vi "ABB Test No Load.vi"() -> ()   [LabVIEW 2017]
uses:
  Temp error msg.ctl
  Video Display Buttons.ctl
  <vilib>/Analysis/baseanly.llb/Mean (DBL).vi
  ABB global.vi
  <vilib>/Analysis/NI_AALPro.lvlib
  <vilib>/Analysis/NI_AALBase.lvlib
panel:
  in  "Video Displays":T1
  in  "Temp error":T2="Error: Temperature measurement "
  in  "Case Constant\n(See Context Help)":i32
  in  "Additional Mech Loss (kW)":dbl
  in  "show fit":bool
  out "Additional Temperatures  (°C)":string[][](table)
  in  "Simulate volts":dbl(slide) max=1800.0
  out "Temperatures  (°C)":string[][](table)
  out "Losses (kW)":string[][](table)
  out "Auto Readings":cluster{"%":dbl[], "Recorded":bool[]}
  out "In Range?":bool[](array[boolean])
  out "saved Readings":dbl[][](array[numeric])
  out "% rated voltage":dbl format="%.1f"
  out "Rated Volts":dbl
  out "Serial number":string
  out "W.O number":string
  out "Power":string[][](table)
  out "Voltage":string[][](table)
  out "Current":string[][](table)
  out "Norma 5000 Error":string
  in  "Record":bool
  out "Readings":string[][](table)
  in  "View":enum16{"Graph", "Readings"}(ring)
  out "Number readings":i32
  out "Status":enum16{"Stopped", "Running"}(ring)
  out "Timedate":string
  in  "End test":bool
  in  "Start":bool
  in  "Read Mode":enum16{"Auto", "Manual"}(ring)
  in  "Exit":bool
  out "Separation of losses":cluster{dbl[], "Best Linear Fit":dbl[]}[](graph)
  # "No Load Test"
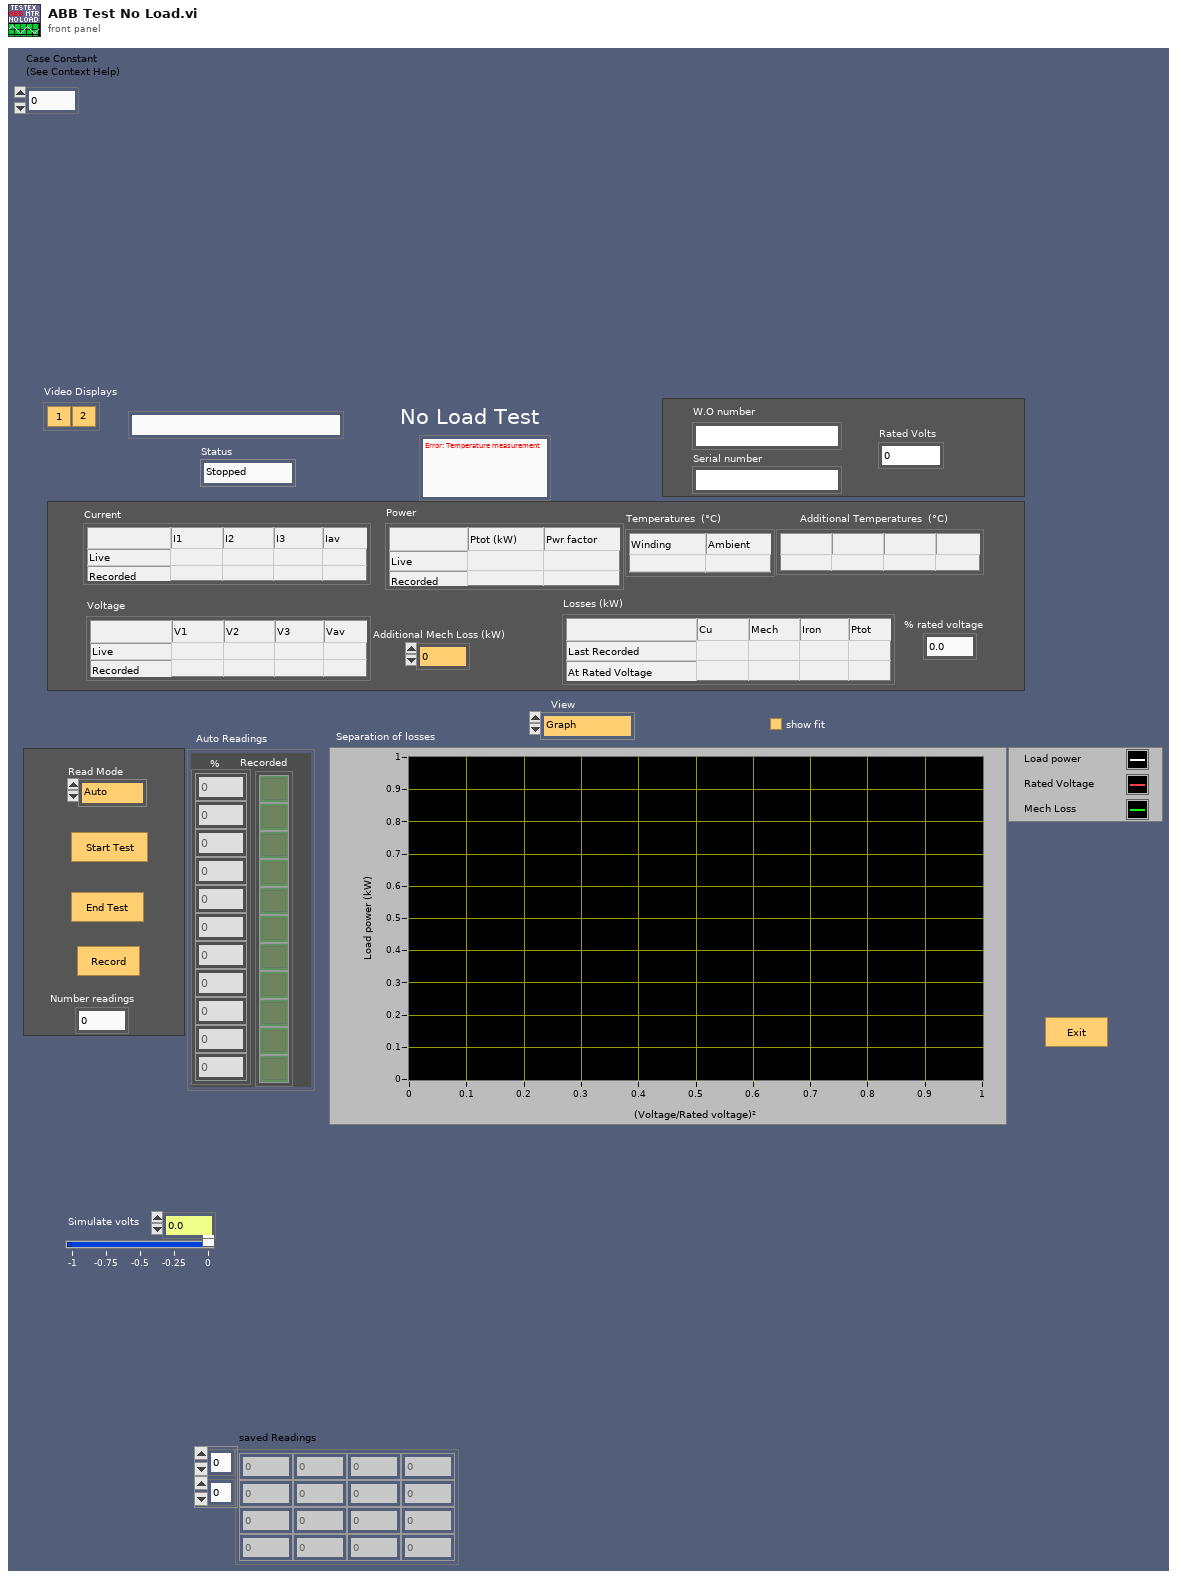
[diagram p1: front panel]
types:
  T1 = typedef "Video Display Buttons.ctl" = cluster{"1":bool, "1 2":bool}
  T2 = typedef "Temp error msg.ctl" = string
  T3 = cluster{"Voltage":dbl, "Current":dbl, "Power":dbl, "power factor":dbl}
  T4 = cluster{"VT Primary":dbl, "VT Secondary":dbl, "CT  Primary":dbl, "CT Secondary":dbl, "Current Shunt":enum16{"Internal", "External"}, "Avg interval":dbl}
  T5 = cluster{"VT Primary":dbl, "VT Secondary":dbl, "CT  Primary":dbl, "CT Secondary":dbl, "Current Shunt":enum16{"Internal", "External"}, "Averaging interval (secs)":dbl}
  T6 = cluster{"Visa sesssion":refnum<visa-resource-name>, "error":errorcluster}
  T7 = cluster{"Simulate Norma":bool, "Norma 5000 Address":u8, "WebDaq IP Address":string, "Simulate cDAQ":bool}
  T8 = cluster{"Number Values":i32, "Tolerance ":dbl, "Value (ratio)":dbl[], "Hold time (sec)":dbl}
  T9 = cluster{"temp. alloc":i32[], "category":i32[], "Category names":string[], "Category none names":string[]}
  T10 = cluster{"PCu":dbl, "Pmech":dbl, "PFe":dbl, "Ptot":dbl, "Ambient":dbl, "I1":dbl, "I2":dbl, "I3":dbl, "Wdg Temp":dbl}
  T11 = cluster{"V":dbl, "A":dbl, "W":dbl, "VA":dbl, "VAr":dbl, "Pf":dbl}
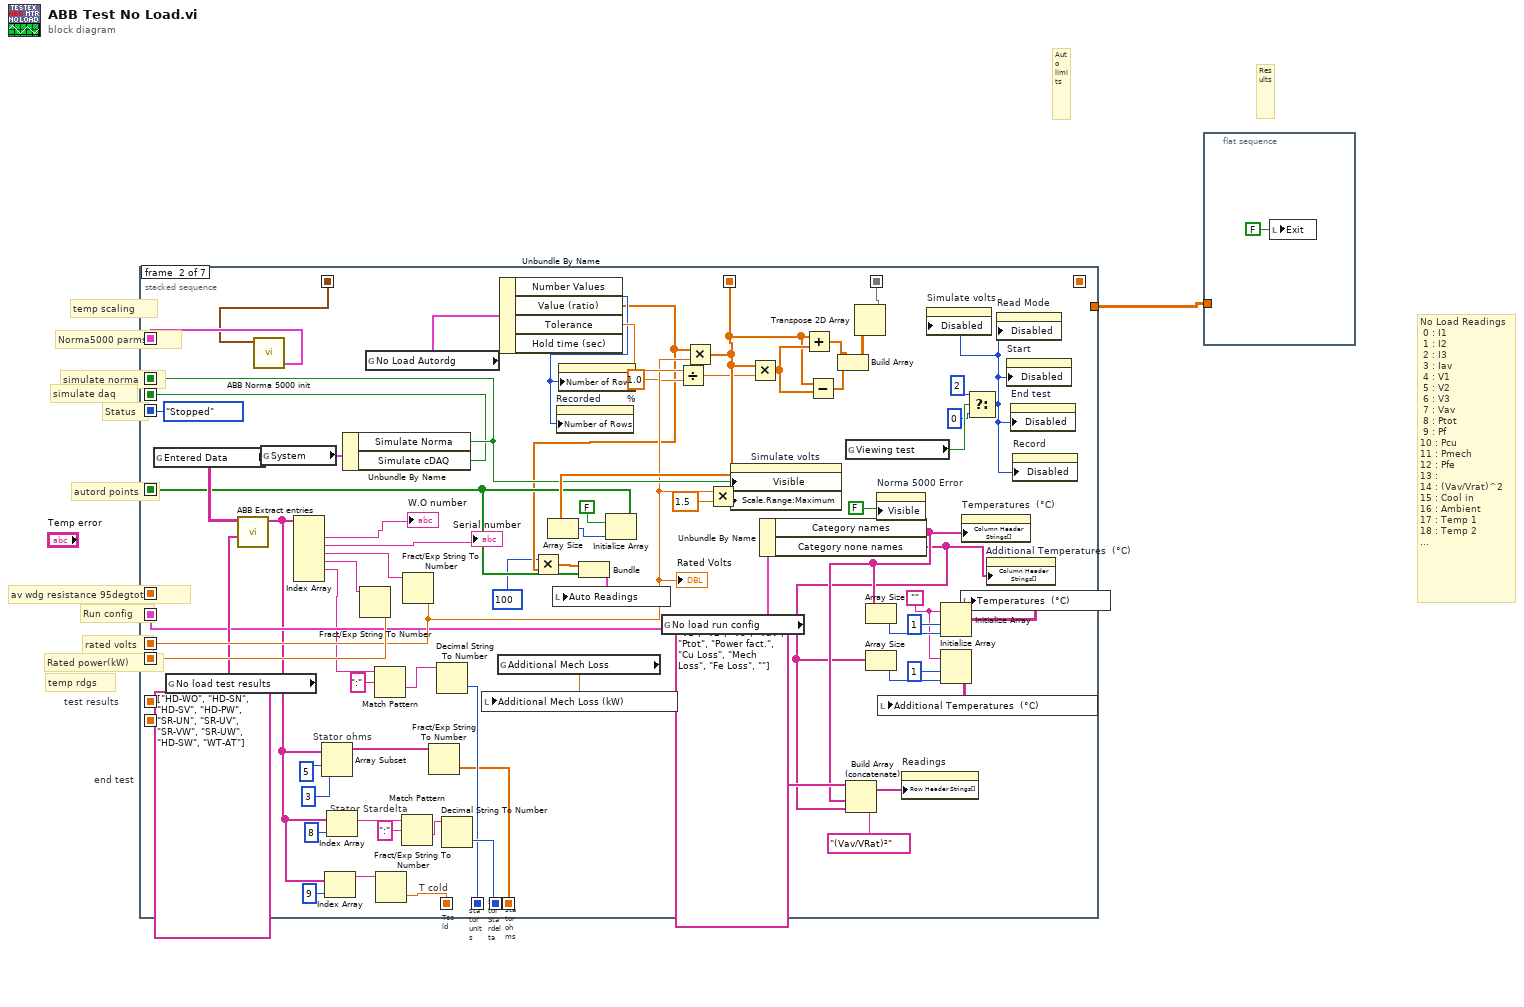
[diagram p0: block diagram]
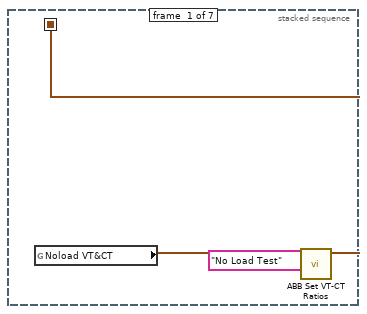
[diagram p2: hidden frame]
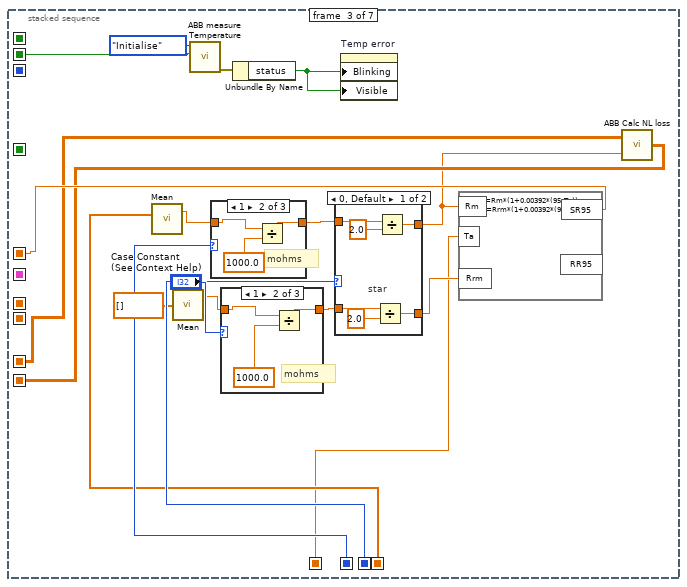
[diagram p3: hidden frame]
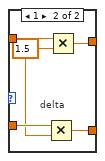
[diagram p4: hidden frame]
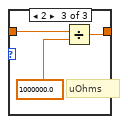
[diagram p6: hidden frame]
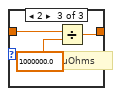
[diagram p8: hidden frame]
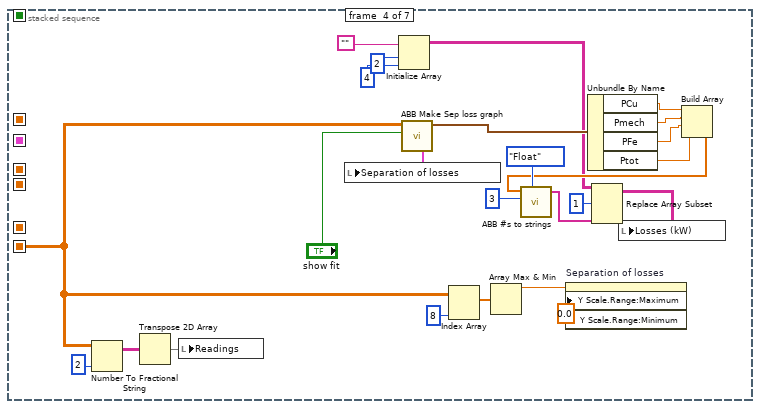
[diagram p9: hidden frame]
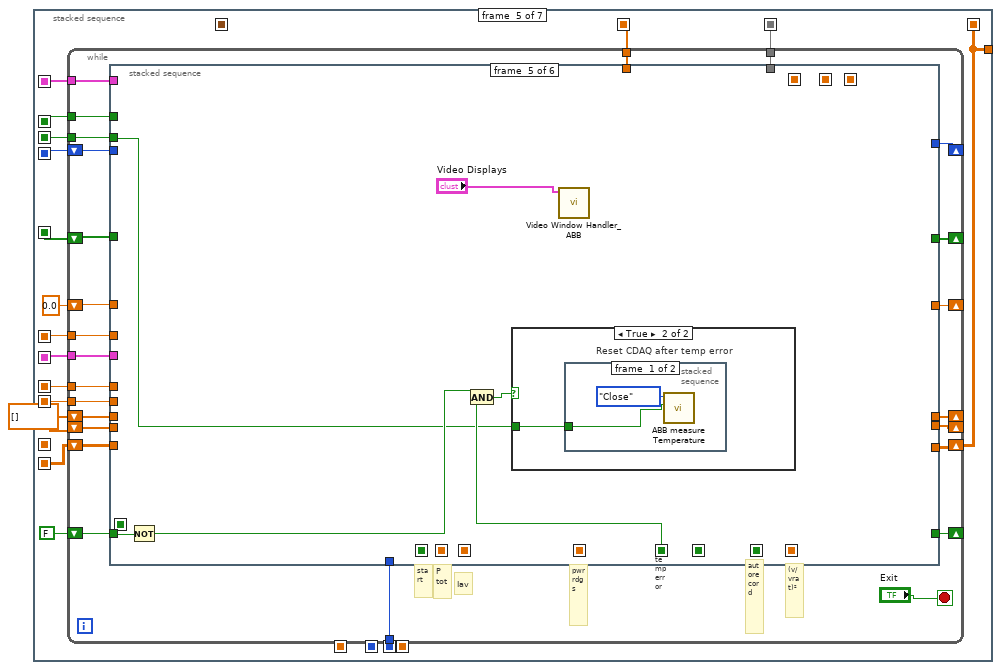
[diagram p10: hidden frame]
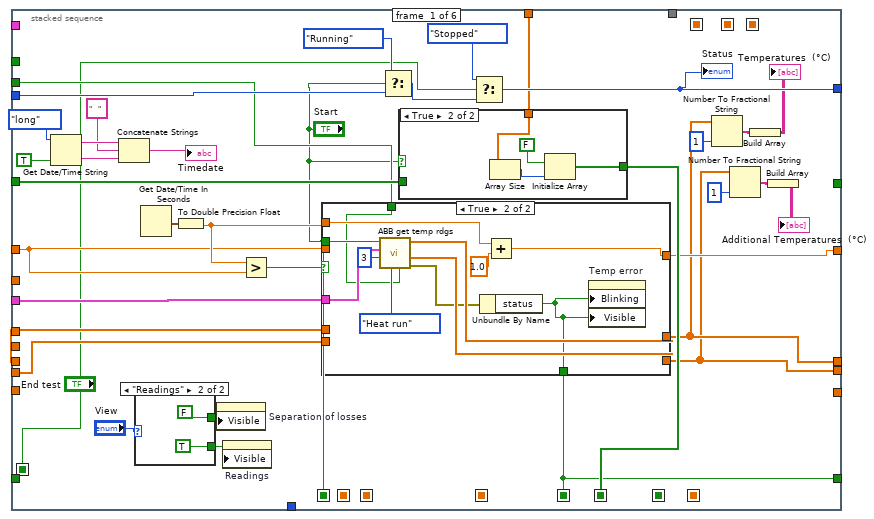
[diagram p11: hidden frame]
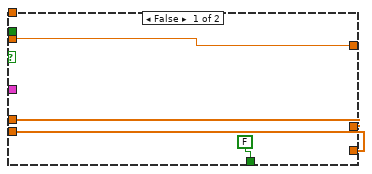
[diagram p12: hidden frame]
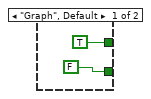
[diagram p14: hidden frame]
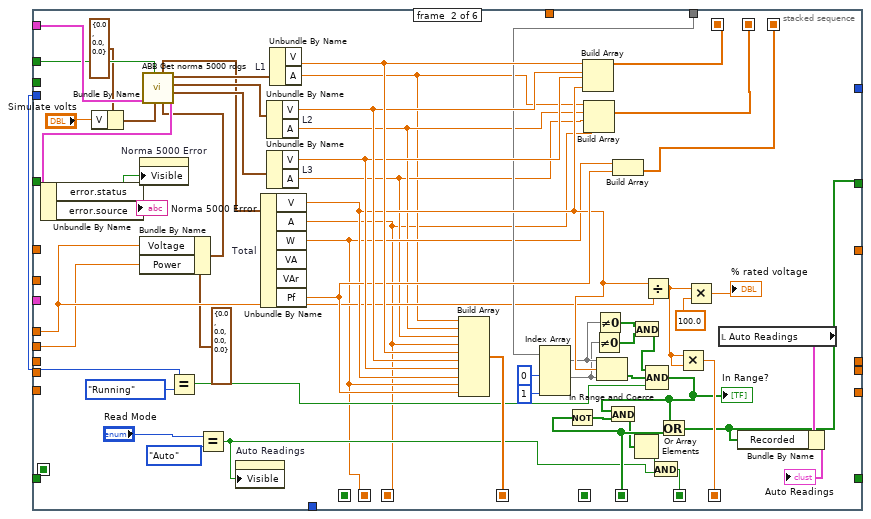
[diagram p15: hidden frame]
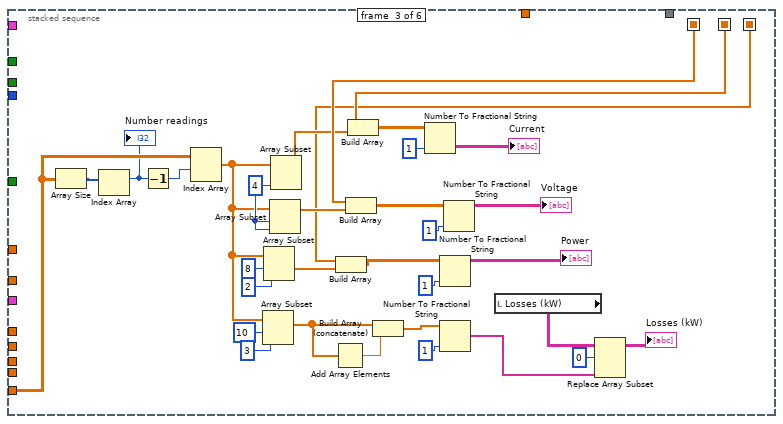
[diagram p16: hidden frame]
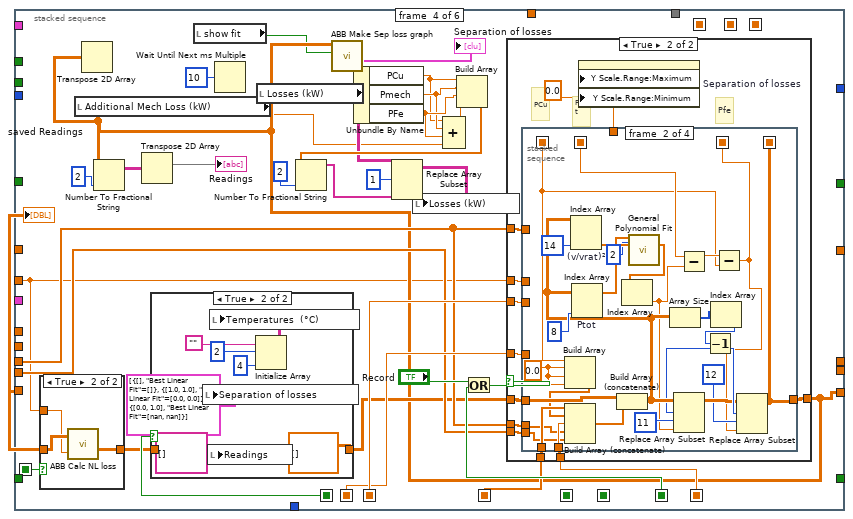
[diagram p17: hidden frame]
diagram:
  # "Results"
  # "Auto limits"
  # "end test"
  # "test results"
  # "stator ohms"
  # "stator units"
  # "Tcold"
  # "Stator Stardelta"
  # "No Load Readings\n 0 : I1\n 1 : I2\n 2 : I3\n 3 : Iav\n 4 : V1\n 5 : V2\n 6 : V3\n 7 : Vav\n 8 : Ptot\n 9 : Pf\n10 : Pcu\n11 : Pmech\n12 : Pfe\n13 :\n14 : (Vav/Vrat)^2\n15 : Cool in\n16 : Ambient\n17 : Temp 1\n18 : Temp 2\n..."
  # "simulate daq"
  # "temp scaling"
  # "temp rdgs"
  # "Run config"
  # "Rated power(kW)"
  # "autord points"
  # "av wdg resistance 95degtot"
  # "rated volts"
  # "simulate norma"
  # "Norma5000 parms"
  # "Status"
  n1 = stacked-sequence {
    seq-local: [_ enum16{"Stopped", "Running"}."Stopped" ("Status") _ _ _ _ _] -> [_ _ _ _ w161 _ _]
    seq-local: [_ w74 _ _ _ _ _] -> [_ _ _ _ w160 w461 _]
    seq-local: [_ w60 _ _ _ _ _] -> [_ _ _ _ w159 w460 _]
    seq-local: [_ w59 _ _ _ _ _] -> [_ _ _ _ w158 _ _]
    seq-local: [_ w47 _ _ _ _ _] -> [_ _ w82 _ _ _ _]
    seq-local: [_ _ w83 _ _ _ _] -> [_ _ _ _ w157 _ _]
    seq-local: [_ w25 _ _ _ _ _] -> [_ _ _ _ w156 _ _]
    seq-local: [_ w66 _ _ _ _ _] -> [_ _ _ _ w154 _ _]
    seq-local: [_ w64 _ _ _ _ _] -> [_ _ _ _ w155 _ _]
    seq-local: [_ w61 _ _ _ _ _] -> [_ _ _ _ w153 _ _]
    seq-local: [_ w27 _ _ _ _ _] -> [_ _ _ _ w151 _ _]
    seq-local: [_ _ _ _ w145 _ _] -> [_ _ _ _ _ w458 _]
    seq-local: [_ w38 _ _ _ _ _] -> [_ _ w79 _ w150 w455 _]
    seq-local: [_ w16 _ _ _ _ _] -> [_ _ w87 _ w148 _ _]
    seq-local: [w2 _ _ _ _ _ _] -> [_ w12 _ _ _ w457 _]
    seq-local: [_ w11 _ _ _ _ _] -> [_ _ w84 _ _ _ _]
    seq-local: [_ w10 _ _ _ _ _] -> [_ _ w88 _ _ _ _]
    seq-local: [_ w9 _ _ _ _ _] -> [_ _ w86 _ _ _ _]
    seq-local: [_ _ w81 _ _ _ _] -> [_ _ _ w121 w147 _ _]
    tunnel: [_ _ _ _ w145 _ _] -> w1
    frame #0 {
      n2 = global read "ABB global.vi" "Noload VT&CT"() -> (w4:T4)
      n3 = call "ABB Set VT-CT Ratios.vi"("Test name"="No Load Test", "VT and CT Ratios"=w4) -> ("VT and CT Ratios out"=w2:T5)  [unwired: 9 in]
    }
    frame #1 {
      w29 = ""
      # "T cold"
      # "Stator Stardelta"
      # "Stator ohms"
      n4 = global read "ABB global.vi" "Entered Data"() -> (w56:string[][])
      n5 = global read "ABB global.vi" "No load test results"() -> (w47:dbl[][])
      n6 = call "ABB Extract entries.vi"("Entry IDs"=string[] ["HD-WO", "HD-SN", "HD-SV", "HD-PW", "SR-UN", "SR-UV", "SR-VW", "SR-UW", "HD-SW", "WT-AT"], "Entry table in"=w56) -> ("Selected Entries"=w14:string[])  [unwired: 9 in]
      n7 = call "ABB Norma 5000 init.vi"("VT and CT Ratios"=w12) -> ("norma 5000 parms out"=w74:T6)  [unwired: 10 in]
      n8 = global read "ABB global.vi" "System"() -> (w73:T7)
      n9 = Index Array(array=w14) -> (element #1=→"W.O number":string, element #2=→"Serial number":string, element #3=w53:string, element #4=w52:string, element #5=w7:string)  [unwired: 6 in, 1 out]
      n10 = Array Subset(array=w14, index=5, length=3) -> (w49:string[])
      n11 = Index Array(array=w14, index=9) -> (element=w13:string)
      n12 = Index Array(array=w14, index=8) -> (element=w19:string)
      n13 = Unbundle By Name(w73) -> ("Simulate Norma"=w60:bool, "Simulate cDAQ"=w38:bool)
      n14 = Fract/Exp String To Number(string=w52) -> (number=w61:dbl)  [unwired: 3 in, 1 out]
      n15 = global read "ABB global.vi" "No Load Autordg"() -> (w63:T8)
      n16 = Match Pattern(string=w7, regular expression=":") -> (after substring=w6:string)  [unwired: 1 in, 3 out]
      n17 = Fract/Exp String To Number(string=w13) -> (number=w11:dbl)  [unwired: 3 in, 1 out]
      n18 = Match Pattern(string=w19, regular expression=":") -> (after substring=w17:string)  [unwired: 1 in, 3 out]
      n19 = Fract/Exp String To Number(string=w53) -> (number=w59:dbl)  [unwired: 3 in, 1 out]
      "Rated Volts" <- w59
      n20 = Fract/Exp String To Number(string=w49) -> (number=w9:dbl[])  [unwired: 3 in, 1 out]
      n21 = Decimal String To Number(string=w6) -> (number=w10:i32)  [unwired: 2 in, 1 out]
      n22 = Decimal String To Number(string=w17) -> (number=w16:i32)  [unwired: 2 in, 1 out]
      n23 = global read "ABB global.vi" "Additional Mech Loss"() -> (w5:dbl)
      n24 = local write "Additional Mech Loss (kW)"(w5) -> ()
      n25 = Unbundle By Name(w63) -> ("Number Values"=w26:i32, "Value (ratio)"=w24:dbl[], "Tolerance"=w62:dbl)  [unwired: 1 out]
      n26 = Multiply(x=100 ("Numeric"), y=w24) -> (x*y=w22:dbl[])
      n27 = property on="Recorded" class="Arr (strict)"("Number of Rows"=w26) -> ()  [unwired: 2 in, 2 out]
      n28 = property on="%" class="Arr (strict)"("Number of Rows"=w26) -> ()  [unwired: 2 in, 2 out]
      n29 = global read "ABB global.vi" "No load run config"() -> (w27:T9)
      n30 = Divide(x=w62, y=1.0) -> (x/y=w46:dbl)
      n31 = Multiply(x=w24, y=w59) -> (x*y=w64:dbl[])
      n32 = Array Size(array=w64) -> (size(s)=w71:i32)
      n33 = Initialize Array(FALSE, w71) -> (w25:bool[])
      n34 = Bundle(w22, w25) -> (w23:cluster{dbl[], bool[]})  [unwired: 1 in]
      n35 = local write "Auto Readings"(w23) -> ()
      n36 = Multiply(x=w59, y=1.5) -> (x*y=w57:dbl)
      n37 = property on="Simulate volts" class="Slide (strict)"("Visible"=w60, "Scale.Range:Maximum"=w57) -> ()  [unwired: 2 in, 2 out]
      n38 = Multiply(x=w64, y=w46) -> (x*y=w68:dbl[])
      n39 = Unbundle By Name(w27) -> ("Category names"=w34:string[], "Category none names"=w31:string[])
      n40 = Add(x=w64, y=w68) -> (x+y=w69:dbl[])
      n41 = Subtract(x=w64, y=w68) -> (x-y=w65:dbl[])
      n42 = Build Array(w69, w65) -> (w67:dbl[][])
      n43 = global read "ABB global.vi" "Viewing test"() -> (w42:bool)
      n44 = Build Array (concatenate)(string[] ["I1", "I2", "I3", "Iav", "V1", "V2", "V3", "Vav", "Ptot", "Power fact.", "Cu Loss", "Mech Loss", "Fe Loss", ""], "(Vav/VRat)²", w34, w31) -> (w43:string[])
      n45 = Transpose 2D Array(2D array=w67) -> (transposed array=w66:dbl[][])
      n46 = Array Size(array=w34) -> (size(s)=w36:i32)
      n47 = Array Size(array=w31) -> (size(s)=w28:i32)
      n48 = property on="Norma 5000 Error" class="Str"("Visible"=FALSE) -> ()  [unwired: 2 in, 2 out]
      n49 = property on="Readings" class="Tbl (strict)"("Row Header Strings[]"=w43) -> ()  [unwired: 2 in, 2 out]
      n50 = Initialize Array(w29, 1 ("dimension size"), w36) -> (w33:string[][])
      n51 = Initialize Array(w29, 1 ("dimension size"), w28) -> (w30:string[][])
      n52 = local write "Additional Temperatures  (°C)"(w30) -> ()
      n53 = local write "Temperatures  (°C)"(w33) -> ()
      n54 = property on="Temperatures  (°C)" class="Tbl (strict)"("Column Header Strings[]"=w34) -> ()  [unwired: 2 in, 2 out]
      n55 = Select(t=2, s=w42, f=0) -> (s? t:f=w39:i32)
      n56 = property on="Simulate volts" class="Slide (strict)"("Disabled"=w39) -> ()  [unwired: 2 in, 2 out]
      n57 = property on="Additional Temperatures  (°C)" class="Tbl (strict)"("Column Header Strings[]"=w31) -> ()  [unwired: 2 in, 2 out]
      n58 = property on="Read Mode" class="Enum (strict)"("Disabled"=w39) -> ()  [unwired: 2 in, 2 out]
      n59 = property on="Start" class="Bool"("Disabled"=w39) -> ()  [unwired: 2 in, 2 out]
      n60 = property on="End test" class="Bool"("Disabled"=w39) -> ()  [unwired: 2 in, 2 out]
      n61 = property on="Record" class="Bool"("Disabled"=w39) -> ()  [unwired: 2 in, 2 out]
    }
    frame #2 {
      n62 = call-poly <vilib>:"Mean.vi"("X"=w86) -> ("mean"=w94:dbl)  [unwired: 1 out]
      n63 = call-poly <vilib>:"Mean.vi"("X"=dbl[] []) -> ("mean"=w92:dbl)  [unwired: 1 out]
      n64 = call "ABB measure Temperature.vi"("Simulate"=w79, "Mode"=enum16{"Initialise", "Read", "Close"}."Initialise") -> ("error out"=w77:errorcluster)  [unwired: 7 in, 2 out]
      n65 = case shown="1" w88 {
        tunnel: w94 -> [w113 w116 w119]
        tunnel: [w113 w114 w117] -> w91
        frame 0, Default {
          # "ohms"
        }
        frame 1 {
          # "mohms"
          n66 = Divide(x=w116, y=1000.0) -> (x/y=w114:dbl)
        }
        frame 2 {
          # "uOhms"
          n67 = Divide(x=w119, y=1000000.0) -> (x/y=w117:dbl)
        }
      }
      n68 = case shown="1" "Case Constant\n(See Context Help)" {
        tunnel: w92 -> [w106 w109 w112]
        tunnel: [w106 w107 w110] -> w90
        frame 0, Default {
          # "ohms"
        }
        frame 1 {
          # "mohms"
          n69 = Divide(x=w109, y=1000.0) -> (x/y=w107:dbl)
        }
        frame 2 {
          # "uOhms"
          n70 = Divide(x=w112, y=1000000.0) -> (x/y=w110:dbl)
        }
      }
      n71 = Unbundle By Name(w77) -> ("status"=w76:bool)
      n72 = case shown="0, Default" w87 {
        tunnel: w91 -> [w100 w105]
        tunnel: [w98 w104] -> w80
        tunnel: w90 -> [w97 w103]
        tunnel: [w96 w102] -> w89
        frame 0, Default {
          # "star"
          n73 = Divide(x=w97, y=2.0) -> (x/y=w96:dbl)
          n74 = Divide(x=w100, y=2.0) -> (x/y=w98:dbl)
        }
        frame 1 {
          w101 = 1.5 ("y")
          # "delta"
          n75 = Multiply(x=w103, y=w101) -> (x*y=w102:dbl)
          n76 = Multiply(x=w105, y=w101) -> (x*y=w104:dbl)
        }
      }
      n77 = property on="Temp error" class="Str (strict)"("Blinking"=w76, "Visible"=w76) -> ()  [unwired: 2 in, 2 out]
      n78 = formula code="SR95=Rm*(1+0.00392*(95-Ta));\nRR95=Rrm*(1+0.00392*(95-Ta));"("Rm"=w80, "Ta"=w84, "Rrm"=w89) -> ("SR95"=w83:dbl)  [unwired: 1 out]
      n79 = call "ABB Calc NL loss.vi"("SR95"=w80, "No load test results 2"=w82) -> ("No load test results"=w81:dbl[][])
    }
    frame #3 {
      n80 = Number To Fractional String(number=w121, precision (6)=i16 2) -> (F-format string=w143:string[][])  [unwired: 2 in]
      n81 = Transpose 2D Array(2D array=w143) -> (transposed array=w142:string[][])
      n82 = local write "Readings"(w142) -> ()
      n83 = Initialize Array("", 2, 4) -> (w126:string[][])
      n84 = call "ABB Make Sep loss graph.vi"("Show fit"="show fit", "Results"=w121) -> ("Sep Loss Graph"=w141:cluster{dbl[], dbl[]}[], "Rated V Readings"=w128:T10)  [unwired: 7 in, 1 out]
      n85 = local write "Separation of losses"(w141) -> ()
      n86 = Index Array(array=w121, index (col)=8 ("disabled index (col)")) -> (element=w124:dbl[])  [unwired: 1 in]
      n87 = Array Max & Min(array=w124) -> (max value=w123:dbl)  [unwired: 3 out]
      n88 = property on="Separation of losses" class="XYGraph (strict)"("Y Scale.Range:Maximum"=w123, "Y Scale.Range:Minimum"=0.0) -> ()  [unwired: 2 in, 2 out]
      n89 = Unbundle By Name(w128) -> ("PCu"=w137:dbl, "Pmech"=w136:dbl, "PFe"=w135:dbl, "Ptot"=w134:dbl)
      n90 = Build Array(w137, w136, w135, w134) -> (w127:dbl[])
      n91 = call "ABB #s to strings.vi"("# type"=enum16{"Float", "Relative time HH:MM"}."Float", "Precision"=3, "Numbers in"=w127) -> ("Strings out"=w129:string[])  [unwired: 8 in]
      n92 = Replace Array Subset(array=w126, new element=w129, index (row)=1) -> (w131:string[][])  [unwired: 1 in]
      n93 = local write "Losses (kW)"(w131) -> ()
    }
    frame #4 {
      w149 = dbl[] []
      n94 = while {
        shift-right: [w184] -> _
        shift-left: w161 -> [w185]
        tunnel: w160 -> [w183]
        tunnel: w159 -> [w182]
        tunnel: w158 -> [w181]
        shift-right: [w179] -> w145
        shift-left: w147 -> [w180]
        tunnel: w157 -> [w178]
        shift-right: [w177] -> _
        shift-left: w156 -> [w176]
        tunnel: w155 -> [w175]
        tunnel: w154 -> [w174]
        tunnel: w153 -> [w173]
        shift-right: [w171] -> _
        shift-left: 0.0 -> [w172]
        tunnel: w151 -> [w170]
        shift-right: [w169] -> _
        shift-left: w149 -> [w168]
        tunnel: w150 -> [w167]
        shift-right: [w165] -> _
        shift-left: w149 -> [w166]
        tunnel: w148 -> [w164]
        shift-right: [w163] -> _
        shift-left: FALSE ("status") -> [w162]
        stop <- "Exit" stop-if-true
        # "temp error"
        # "P tot"
        # "Iav"
        # "autorecord"
        # "(v/vrat)²"
        # "pwr rdgs"
        # "start"
        n95 = stacked-sequence {
          seq-local: ["Start" _ _ _ _ _] -> [_ _ _ w373 _ _]
          seq-local: [_ w291 _ _ _ _] -> [_ _ _ w368 _ _]
          seq-local: [_ w289 _ _ _ _] -> [_ _ _ w367 _ _]
          seq-local: [w207 _ _ _ _ _] -> [_ w284 _ _ _ _]
          seq-local: [_ w279 _ _ _ _] -> [_ _ _ w370 _ _]
          seq-local: [_ w275 _ _ _ _] -> [_ _ w332 _ _ _]
          seq-local: [_ w274 _ _ _ _] -> [_ _ w328 _ _ _]
          seq-local: [_ w273 _ _ _ _] -> [_ _ w320 _ _ _]
          seq-local: [_ w249 _ _ _ _] -> [_ _ _ w366 _ _]
          seq-local: [_ w258 _ _ _ _] -> [_ _ _ w365 _ _]
          seq-local: ["End test" _ _ _ _ _] -> [_ _ _ w343 _ _]
          seq-local: [w187 _ _ _ _ _] -> [_ _ _ _ w447 _]
          tunnel: w185 -> [w217 w261 _ _ _ _]
          tunnel: [w213 _ _ _ _ _] -> w184
          tunnel: w183 -> [_ w306 _ _ _ _]
          tunnel: w182 -> [_ w298 _ _ _ _]
          tunnel: w181 -> [_ w272 _ _ _ _]
          tunnel: w180 -> [_ _ w338 w344 _ _]
          tunnel: [_ _ _ w346 _ _] -> w179
          tunnel: w178 -> [_ _ _ w342 _ _]
          tunnel: [_ w254 _ _ _ _] -> w177
          tunnel: w176 -> [w209 _ _ _ _ _]
          tunnel: w175 -> [w208 _ _ _ _ _]
          tunnel: w174 -> [_ w287 _ _ _ _]
          tunnel: w173 -> [_ w256 _ _ _ _]
          tunnel: w172 -> [w202 _ _ _ _ _]
          tunnel: [w203 _ _ _ _ _] -> w171
          tunnel: w170 -> [w201 _ _ _ _ _]
          tunnel: [w196 _ _ _ _ _] -> w169
          tunnel: w168 -> [w200 _ _ w364 _ _]
          tunnel: w167 -> [w199 _ _ _ w444 _]
          tunnel: w166 -> [w198 _ _ w363 _ _]
          tunnel: [w190 _ _ _ _ _] -> w165
          tunnel: w164 -> [_ _ _ _ _ _]
          tunnel: [w187 _ _ _ _ _] -> w163
          tunnel: w162 -> [_ _ _ _ w446 _]
          frame #0 {
            n96 = Get Date/Time String(date format (0)=enum16{"short", "long", "abbreviated"}."long", want seconds? (F)=TRUE) -> (date string=w221:string, time string=w220:string)  [unwired: 1 in]
            n97 = Concatenate Strings(w221, "   ", w220) -> (→"Timedate":string)
            n98 = case shown="\"Readings\"" "View" {
              tunnel: [TRUE FALSE] -> w211
              tunnel: [FALSE TRUE] -> w210
              frame "Graph", Default {
              }
              frame "Readings" {
              }
            }
            n99 = Get Date/Time In Seconds() -> (seconds since 1Jan1904=w205:timestamp)
            n100 = To Double Precision Float(number=w205) -> (double precision float=w204:dbl)
            n101 = property on="Separation of losses" class="XYGraph (strict)"("Visible"=w211) -> ()  [unwired: 2 in, 2 out]
            n102 = property on="Readings" class="Tbl (strict)"("Visible"=w210) -> ()  [unwired: 2 in, 2 out]
            n103 = Greater?(x=w204, y=w202) -> (0:w206:bool)
            n104 = case shown="True" w206 {
              tunnel: w204 -> [_ w239]
              tunnel: [w227 w237] -> w203
              tunnel: w202 -> [w227 _]
              tunnel: w199 -> [_ w230]
              tunnel: w201 -> [_ w236]
              tunnel: [w226 w235] -> w196
              tunnel: w200 -> [w226 _]
              tunnel: w198 -> [w225 _]
              tunnel: [w225 w234] -> w190
              tunnel: "Start" -> [_ w233]
              tunnel: [FALSE ("status") w228] -> w187
              frame False {
              }
              frame True {
                n105 = call "ABB get temp rdgs.vi"("Sim daq"=w230, "sim type"=enum16{"Heat run", "Bearing run"}."Heat run", "# categories"=3, "run config"=w236, "start"=w233) -> ("error out"=w229:errorcluster, "Category none rdgs"=w234:dbl[], "Category rdgs"=w235:dbl[])  [unwired: 3 in, 1 out]
                n106 = Unbundle By Name(w229) -> ("status"=w228:bool)
                n107 = Add(x=w239, y=1.0) -> (x+y=w237:dbl)
                n108 = property on="Temp error" class="Str (strict)"("Blinking"=w228, "Visible"=w228) -> ()  [unwired: 2 in, 2 out]
              }
            }
            n109 = Select(t=enum16{"Stopped", "Running"}."Running", s="Start", f=w217) -> (s? t:f=w215:enum16{"Stopped", "Running"})
            n110 = case shown="True" "Start" {
              tunnel: w208 -> [_ w244]
              tunnel: [w240 w241] -> w207
              tunnel: w209 -> [w240 _]
              frame False {
              }
              frame True {
                n111 = Array Size(array=w244) -> (size(s)=w243:i32)
                n112 = Initialize Array(FALSE, w243) -> (w241:bool[])
              }
            }
            n113 = Select(t=enum16{"Stopped", "Running"}."Stopped", s="End test", f=w215) -> (s? t:f=w213:enum16{"Stopped", "Running"})
            "Status" <- w213
            n114 = Number To Fractional String(number=w196, precision (6)=i16 1) -> (F-format string=w194:string[])  [unwired: 2 in]
            n115 = Number To Fractional String(number=w190, precision (6)=i16 1) -> (F-format string=w192:string[])  [unwired: 2 in]
            n116 = Build Array(w194) -> (→"Temperatures  (°C)":string[][])
            n117 = Build Array(w192) -> (→"Additional Temperatures  (°C)":string[][])
          }
          frame #1 {
            n118 = Bundle By Name(cluster=cluster{"V":dbl, "A":dbl, "pwr factor":dbl} {"V"=0.0, "A"=0.0, "pwr factor"=0.0} ("Simulation rdgs"), "V"="Simulate volts") -> (w268:cluster{"V":dbl, "A":dbl, "pwr factor":dbl})
            n119 = Bundle By Name(cluster=T3 {"Voltage"=0.0, "Current"=0.0, "Power"=0.0, "power factor"=0.0} ("Rated"), "Voltage"=w272, "Power"=w256) -> (w271:T3)
            n120 = call "ABB Get norma 5000 rdgs.vi"("Rated"=w271, "Simulation rdgs"=w268, "simulate"=w298, "norma 5000 parms in"=w306) -> ("norma 5000 parms out"=w300:T6, "L 3"=w301:T11, "L 2"=w302:T11, "L1"=w303:T11, "Total"=w299:T11)  [unwired: 3 in]
            n121 = Unbundle By Name(w300) -> ("error.status"=w305:bool, "error.source"=→"Norma 5000 Error":string)
            n122 = property on="Norma 5000 Error" class="Str"("Visible"=w305) -> ()  [unwired: 2 in, 2 out]
            n123 = Equal?(x=w261, y=enum16{"Stopped", "Running"}."Running") -> (x = y?=w259:bool)
            n124 = Equal?(x="Read Mode", y=enum16{"Auto", "Manual"}."Auto") -> (x = y?=w276:bool)
            n125 = property on="Auto Readings" class="Clust (strict)"("Visible"=w276) -> ()  [unwired: 2 in, 2 out]
            n126 = Unbundle By Name "Total"(w299) -> ("V"=w288:dbl, "A"=w249:dbl, "W"=w258:dbl, "Pf"=w292:dbl)  [unwired: 2 out]
            n127 = Unbundle By Name "L2"(w302) -> ("V"=w294:dbl, "A"=w252:dbl)
            n128 = Unbundle By Name "L3"(w301) -> ("V"=w293:dbl, "A"=w251:dbl)
            n129 = Unbundle By Name "L1"(w303) -> ("V"=w295:dbl, "A"=w250:dbl)
            n130 = Build Array(w250, w252, w251, w249, w295, w294, w293, w288, w258, w292) -> (w291:dbl[])
            n131 = Index Array(array=w287, index (col) #1=0 ("disabled index (col)"), index (col) #2=1 ("index (col)")) -> (element #1=w267:dbl[], element #2=w266:dbl[])  [unwired: 2 in]
            n132 = Not(x=w284) -> (.not. x?=w282:bool[])
            n133 = Build Array(w295, w294, w293, w288) -> (w275:dbl[])
            n134 = Build Array(w250, w252, w251, w249) -> (w274:dbl[])
            n135 = Not Equal To 0?(x=w266) -> (x != 0?=w264:bool[])
            n136 = Not Equal To 0?(x=w267) -> (x != 0?=w265:bool[])
            n137 = In Range and Coerce(upper limit=w267, x=w288, lower limit=w266) -> (In Range?=w283:bool[])  [unwired: 1 out]
            n138 = Build Array(w258, w292) -> (w273:dbl[])
            n139 = And(x=w265, y=w264) -> (x .and. y?=w262:bool[])
            n140 = Divide(x=w288, y=w272) -> (x/y=w290:dbl)
            n141 = Compound Arithmetic op=AND(w262, w283, w259) -> (w263:bool[])
            "In Range?" <- w263
            n142 = And(x=w263, y=w282) -> (x .and. y?=w281:bool[])
            n143 = Or Array Elements(Boolean array=w281) -> (logical OR=w280:bool)
            n144 = And(x=w280, y=w276) -> (x .and. y?=w279:bool)
            n145 = Or(x=w263, y=w284) -> (x .or. y?=w254:bool[])
            n146 = Multiply(x=w290, y=w290) -> (x*y=w289:dbl)
            n147 = Multiply(x=w290, y=100.0) -> (x*y=→"% rated voltage":dbl)
            n148 = local read "Auto Readings"() -> (w255:cluster{"%":dbl[], "Recorded":bool[]})
            n149 = Bundle By Name(cluster=w255, "Recorded"=w254) -> (→"Auto Readings":cluster{"%":dbl[], "Recorded":bool[]})
          }
          frame #2 {
            w335 = 4 ("length")
            n150 = Array Size(array=w338) -> (size(s)=w339:i32[])
            n151 = Index Array(array=w339) -> (element=w314:i32)  [unwired: 1 in]
            "Number readings" <- w314
            n152 = Decrement(x=w314) -> (x-1=w337:i32)
            n153 = Index Array(array=w338, index (row)=w337) -> (element=w317:dbl[])  [unwired: 1 in]
            n154 = Array Subset(array=w317, index=10, length=3) -> (w309:dbl[])
            n155 = Array Subset(array=w317, index=8, length=2) -> (w321:dbl[])
            n156 = Array Subset(array=w317, index=w335, length=w335) -> (w334:dbl[])
            n157 = Array Subset(array=w317, length=w335) -> (w327:dbl[])  [unwired: 1 in]
            n158 = Add Array Elements(numeric array=w309) -> (sum=w307:dbl)
            n159 = Build Array(w320, w321) -> (w322:dbl[][])
            n160 = Build Array(w332, w334) -> (w333:dbl[][])
            n161 = Build Array(w328, w327) -> (w326:dbl[][])
            n162 = Build Array (concatenate)(w309, w307) -> (w308:dbl[])
            n163 = Number To Fractional String(number=w326, precision (6)=i16 1) -> (F-format string=→"Current":string[][])  [unwired: 2 in]
            n164 = Number To Fractional String(number=w322, precision (6)=i16 1) -> (F-format string=→"Power":string[][])  [unwired: 2 in]
            n165 = Number To Fractional String(number=w308, precision (6)=i16 1) -> (F-format string=w310:string[])  [unwired: 2 in]
            n166 = Number To Fractional String(number=w333, precision (6)=i16 1) -> (F-format string=→"Voltage":string[][])  [unwired: 2 in]
            n167 = local read "Losses (kW)"() -> (w313:string[][])
            n168 = Replace Array Subset(array=w313, new element=w310, index (row)=0) -> (→"Losses (kW)":string[][])  [unwired: 1 in]
          }
          frame #3 {
            n169 = case shown="True" w343 {
              tunnel: [w374 w376] -> w345
              tunnel: w344 -> [w374 w377]
              tunnel: w342 -> [_ w375]
              frame False {
              }
              frame True {
                n170 = call "ABB Calc NL loss.vi"("SR95"=w375, "No load test results 2"=w377) -> ("No load test results"=w376:dbl[][])
              }
            }
            n171 = local read "Additional Mech Loss (kW)"() -> (w340:dbl)
            n172 = case shown="True" w373 {
              tunnel: w345 -> [w378 _]
              tunnel: [w378 dbl[][] []] -> w362
              frame False {
              }
              frame True {
                n173 = local write "Separation of losses"(cluster{dbl[], "Best Linear Fit":dbl[]}[] [{[], "Best Linear Fit"=[]}, {[1.0, 1.0], "Best Linear Fit"=[0.0, 0.0]}, {[0.0, 1.0], "Best Linear Fit"=[nan, nan]}] ("Separation of losses")) -> ()
                n174 = local write "Readings"(string[][] [] ("Readings")) -> ()
                n175 = Initialize Array("", 2 ("dimension size"), 4 ("dimension size")) -> (w379:string[][])
                n176 = local write "Temperatures  (°C)"(w379) -> ()
              }
            }
            n177 = local read "show fit"() -> (w341:bool)
            n178 = Wait Until Next ms Multiple(millisecond multiple=u32 10) -> ()  [unwired: 1 out]
            n179 = local read "Losses (kW)"() -> (w352:string[][])
            n180 = Or(x="Record", y=w370) -> (x .or. y?=w371:bool)
            n181 = case shown="True" w371 {
              tunnel: w362 -> [w386 w398]
              tunnel: [w386 w397] -> w346
              tunnel: w368 -> [_ w396]
              tunnel: w364 -> [_ w395]
              tunnel: w367 -> [_ w394]
              tunnel: w342 -> [_ w393]
              tunnel: w366 -> [_ w392]
              tunnel: w364 -> [_ w391]
              tunnel: w365 -> [_ w390]
              tunnel: w363 -> [_ w387]
              frame False {
              }
              frame True {
                # "Pfe"
                # "Ptot"
                # "PCu"
                n182 = stacked-sequence {
                  seq-local: [w402 _ _ _] -> [_ w410 _ _]
                  seq-local: [w400 _ _ _] -> [_ w424 _ _]
                  seq-local: [_ w412 _ _] -> [_ _ _ _]
                  seq-local: [_ w416 _ _] -> [_ _ w440 _]
                  tunnel: w398 -> [_ w432 _ _]
                  tunnel: [_ w416 _ _] -> w397
                  tunnel: w396 -> [_ w430 _ _]
                  tunnel: w395 -> [_ w414 w434 _]
                  tunnel: w394 -> [_ w415 _ _]
                  tunnel: w393 -> [w405 _ _ _]
                  tunnel: w392 -> [w404 _ _ _]
                  tunnel: w391 -> [_ _ _ _]
                  tunnel: w390 -> [w400 _ _ _]
                  tunnel: [_ _ w439 _] -> w388
                  tunnel: w387 -> [_ w413 _ _]
                  frame #0 {
                    # "Cu loss = Iav*Iav*R95tot"
                    n183 = Compound Arithmetic op=MULTIPLY(w405, w404, w404, 3.0 ("value")) -> (w403:dbl)
                    n184 = Divide(x=w403, y=1000.0) -> (x/y=w402:dbl)
                  }
                  frame #1 {
                    w409 = 0.0 ("element")
                    n185 = Build Array(w410, w409, w409, w409) -> (w428:dbl[])
                    n186 = Build Array (concatenate)(w430, w428, w415, w414, w413) -> (w431:dbl[])
                    n187 = Build Array (concatenate)(w432, w431) -> (w423:dbl[][])
                    n188 = Index Array "(v/vrat)²"(array=w423, index (col)=14 ("disabled index (col)")) -> (element=w425:dbl[])  [unwired: 1 in]
                    n189 = Index Array "Ptot"(array=w423, index (col)=8 ("disabled index (col)")) -> (element=w426:dbl[])  [unwired: 1 in]
                    n190 = call <vilib>:"General Polynomial Fit.vi"("Y"=w426, "polynomial order"=2, "X"=w425) -> ("Polynomial Coefficients"=w407:dbl[])  [unwired: 9 in, 3 out]
                    n191 = Index Array(array=w407) -> (element=w406:dbl)  [unwired: 1 in]
                    n192 = Array Size(array=w423) -> (size(s)=w422:i32[])
                    n193 = Subtract(x=w424, y=w406) -> (x-y=w411:dbl)
                    n194 = Index Array(array=w422) -> (element=w421:i32)  [unwired: 1 in]
                    n195 = Decrement(x=w421) -> (x-1=w420:i32)
                    n196 = Replace Array Subset(array=w423, new element=w406, index (row)=w420, index (col)=11) -> (w419:dbl[][])
                    n197 = Subtract(x=w411, y=w410) -> (x-y=w412:dbl)
                    n198 = Replace Array Subset(array=w419, new element=w412, index (row)=w420, index (col)=12) -> (w416:dbl[][])
                  }
                  frame #2 {
                    n199 = Index Array(array=w440, index (col)=8 ("disabled index (col)")) -> (element=w441:dbl[])  [unwired: 1 in]
                    n200 = Number To Fractional String(number=w434, precision (6)=i16 1) -> (F-format string=w435:string[])  [unwired: 2 in]
                    n201 = Array Max & Min(array=w441) -> (max value=w439:dbl)  [unwired: 3 out]
                    n202 = local read "Temperatures  (°C)"() -> (w438:string[][])
                    n203 = Replace Array Subset(array=w438, new element=w435, index (row)=1) -> (w437:string[][])  [unwired: 1 in]
                    n204 = local write "Temperatures  (°C)"(w437) -> ()
                  }
                  frame #3 {
                  }
                }
                n205 = property on="Separation of losses" class="XYGraph (strict)"("Y Scale.Range:Maximum"=w388, "Y Scale.Range:Minimum"=0.0) -> ()  [unwired: 2 in, 2 out]
              }
            }
            n206 = Transpose 2D Array(2D array=w346) -> ()  [unwired: 1 out]
            n207 = Number To Fractional String(number=w346, precision (6)=i16 2) -> (F-format string=w349:string[][])  [unwired: 2 in]
            n208 = Transpose 2D Array(2D array=w349) -> (transposed array=→"Readings":string[][])
            n209 = call "ABB Make Sep loss graph.vi"("Show fit"=w341, "Results"=w346) -> ("Sep Loss Graph"=→"Separation of losses":cluster{dbl[], dbl[]}[], "Rated V Readings"=w351:T10)  [unwired: 7 in, 1 out]
            n210 = Unbundle By Name(w351) -> ("PCu"=w356:dbl, "Pmech"=w357:dbl, "PFe"=w358:dbl)
            n211 = Compound Arithmetic op=ADD(w356, w357, w358, w340) -> (w359:dbl)
            n212 = Build Array(w356, w357, w358, w359) -> (w360:dbl[])
            n213 = Number To Fractional String(number=w360, precision (6)=2 ("Precision")) -> (F-format string=w355:string[])  [unwired: 2 in]
            n214 = Replace Array Subset(array=w352, new element=w355, index (row)=1) -> (w353:string[][])  [unwired: 1 in]
            n215 = local write "Losses (kW)"(w353) -> ()
            "saved Readings" <- w344
          }
          frame #4 {
            n216 = Not(x=w446) -> (.not. x?=w445:bool)
            n217 = And(x=w445, y=w447) -> (x .and. y?=w448:bool)
            n218 = case shown="True" w448 {
              tunnel: w444 -> [_ w449]
              frame False {
              }
              frame True {
                # "Reset CDAQ after temp error"
                n219 = stacked-sequence {
                  tunnel: w449 -> [w450 w452]
                  frame #0 {
                    n220 = call "ABB measure Temperature.vi"("Simulate"=w450, "Mode"=enum16{"Initialise", "Read", "Close"}."Close") -> ()  [unwired: 7 in, 3 out]
                  }
                  frame #1 {
                    n221 = call "ABB measure Temperature.vi"("Simulate"=w452, "Mode"=enum16{"Initialise", "Read", "Close"}."Initialise") -> ()  [unwired: 7 in, 3 out]
                  }
                }
              }
            }
            n222 = call "Video Window Handler_ABB.vi"("Video Displays"="Video Displays") -> ()  [unwired: 11 in]
          }
          frame #5 {
            n223 = Wait (ms)(milliseconds to wait=u32 20) -> ()  [unwired: 1 out]
          }
        }
      }
    }
    frame #5 {
      n224 = case shown="False" w460 {
        tunnel: w461 -> [w479 _]
        frame False {
          n225 = Unbundle By Name(w479) -> ("Visa sesssion"=w478:refnum<visa-resource-name>, "error"=w477:errorcluster)
          n226 = call "LNOPA01 Error Query.vi"("error in (no error)"=w477, "VISA session"=w478) -> ("error out"=w480:errorcluster, "dup VISA session"=w481:refnum<visa-resource-name>)  [unwired: 6 in, 2 out]
          n227 = call "LNOPA01 Close.vi"("error in (no error)"=w480, "VISA session"=w481) -> ("error out"=w482:errorcluster)  [unwired: 9 in]
          n228 = call <vilib>:"Simple Error Handler.vi"("error in (no error)"=w482) -> ()  [unwired: 4 in, 5 out]
        }
        frame True {
        }
      }
      n229 = call "ABB measure Temperature.vi"("Simulate"=w455, "Mode"=enum16{"Initialise", "Read", "Close"}."Close") -> ()  [unwired: 7 in, 3 out]
      n230 = global read "ABB global.vi" "Viewing test"() -> (w459:bool)
      n231 = case shown="False" w459 {
        tunnel: w458 -> [w466 _]
        tunnel: w457 -> [w462 _]
        frame False {
          n232 = global read "ABB global.vi" "Current test"() -> (w465:path)
          n233 = Two Button Dialog(message="Save results?", 1:"Discard" ("F button name (\"Cancel\")"), 2:"Save" ("T button name (\"OK\")")) -> (T button?=w467:bool)
          n234 = case shown="True" w467 {
            tunnel: w466 -> [_ w471]
            tunnel: w465 -> [_ w470]
            tunnel: w462 -> [_ w469]
            frame False {
            }
            frame True {
              n235 = stacked-sequence {
                tunnel: w471 -> [w474 _]
                tunnel: w470 -> [_ w475]
                tunnel: w469 -> [w473 _]
                frame #0 {
                  n236 = global write "ABB global.vi" "No load test results"(w474) -> ()
                  n237 = global write "ABB global.vi" "Noload VT&CT"(w473) -> ()
                  n238 = global write "ABB global.vi" "Additional Mech Loss"("Additional Mech Loss (kW)") -> ()
                }
                frame #1 {
                  n239 = call "ABB Load-Save results.vi"("Path"=w475, "Mode"=enum16{"LOAD", "Save"}."Save") -> ()  [unwired: 10 in]
                }
              }
            }
          }
        }
        frame True {
        }
      }
    }
    frame #6 {
      n240 = Wait (ms)(milliseconds to wait=u32 100) -> ()  [unwired: 1 out]
    }
  }
  n241 = flat-sequence {
    tunnel: w1 -> [_]
    frame #0 {
      n242 = local write "Exit"(FALSE ("Exit")) -> ()
    }
  }
